vi "String - EditPos Cluster to String.vi"(11 "EditPos":T1) -> (3 "result string":string)   [LabVIEW 2013]
uses:
  <vilib>/Utility/miscctls.llb/LVRowAndColumnTypeDef.ctl
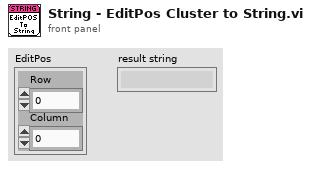
[diagram p1: front panel]
types:
  T1 = typedef "LVRowAndColumnTypeDef.ctl" = cluster{"Row":i32, "Column":i32}
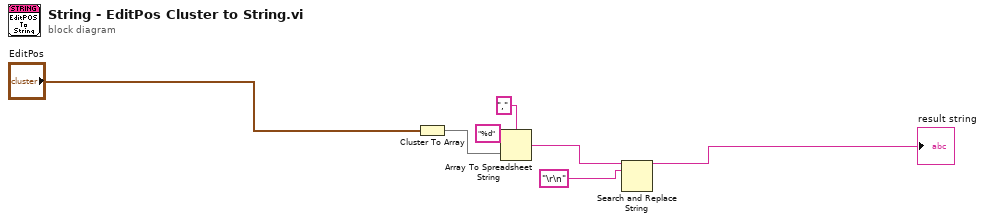
[diagram p0: block diagram]
diagram:
  n1 = Cluster To Array(cluster="EditPos") -> (array=w3:i32[])
  n2 = Array To Spreadsheet String(delimiter (Tab)=",", array=w3, 3:"%d" ("format string")) -> (spreadsheet string=w6:string)
  n3 = Search and Replace String(input string=w6, search string="\r\n" ("input string")) -> (result string=→"result string":string)  [unwired: 6 in, 3 out]
